vi "例程06-初级计算器.vi"() -> ()   [LabVIEW 2018]
panel:
  in  "/":bool
  in  "*":bool
  in  "-":bool
  in  "+":bool
  out "结果":dbl
  in  "输入2":dbl
  in  "输入1":dbl
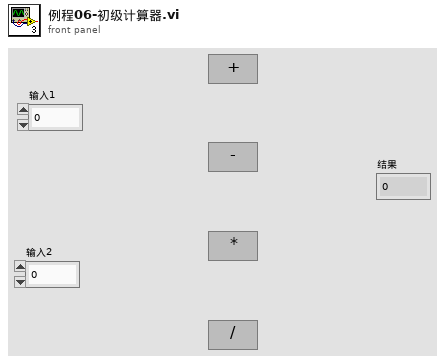
[diagram p1: front panel]
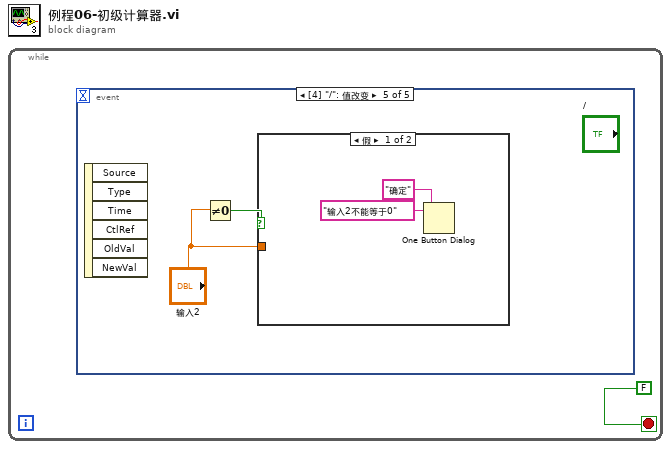
[diagram p0: block diagram]
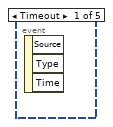
[diagram p2: hidden frame]
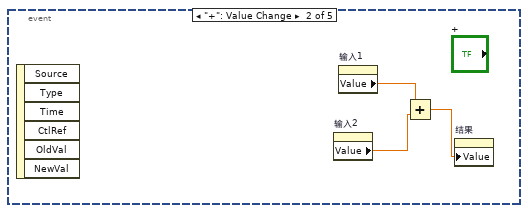
[diagram p3: hidden frame]
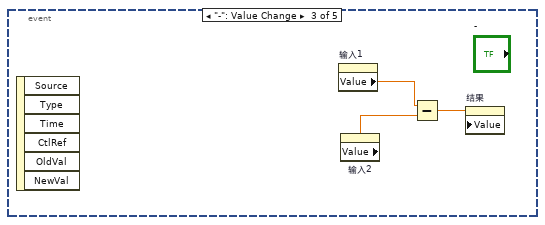
[diagram p4: hidden frame]
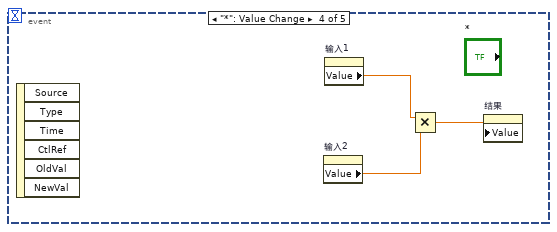
[diagram p5: hidden frame]
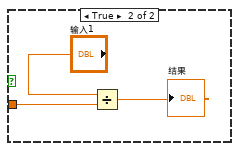
[diagram p6: hidden frame]
diagram:
  n1 = while {
    stop <- FALSE stop-if-true
    n2 = event shown="[4] \"/\": 值改变" {
      selector: _ -> [_ _ _ _ _]
      dyn-events: _ -> [_ _ _ _ _]
      timeout: _ -> [_ _ _ _ _]
      event Timeout {
        n3 = event-data() -> ()  [unwired: 1 in, 3 out]
      }
      event "+": Value Change {
        n4 = event-data() -> ()  [unwired: 1 in, 6 out]
        n5 = property on="输入2" class="DigNum (严格)"() -> ("Value"=w3:dbl)  [unwired: 2 in, 2 out]
        n6 = property on="输入1" class="DigNum (严格)"() -> ("Value"=w4:dbl)  [unwired: 2 in, 2 out]
        n7 = Add(x=w4, y=w3) -> (x+y=w2:dbl)
        n8 = property on="结果" class="DigNum (严格)"("Value"=w2) -> ()  [unwired: 2 in, 2 out]
      }
      event "-": Value Change {
        n9 = event-data() -> ()  [unwired: 1 in, 6 out]
        n10 = property on="输入1" class="DigNum (严格)"() -> ("Value"=w7:dbl)  [unwired: 2 in, 2 out]
        n11 = property on="输入2" class="DigNum (严格)"() -> ("Value"=w6:dbl)  [unwired: 2 in, 2 out]
        n12 = Subtract(x=w7, y=w6) -> (x-y=w5:dbl)
        n13 = property on="结果" class="DigNum (严格)"("Value"=w5) -> ()  [unwired: 2 in, 2 out]
      }
      event "*": Value Change {
        n14 = event-data() -> ()  [unwired: 1 in, 6 out]
        n15 = property on="输入2" class="DigNum (严格)"() -> ("Value"=w9:dbl)  [unwired: 2 in, 2 out]
        n16 = property on="输入1" class="DigNum (严格)"() -> ("Value"=w10:dbl)  [unwired: 2 in, 2 out]
        n17 = Multiply(x=w10, y=w9) -> (x*y=w8:dbl)
        n18 = property on="结果" class="DigNum (严格)"("Value"=w8) -> ()  [unwired: 2 in, 2 out]
      }
      event "/": Value Change {
        n19 = event-data() -> ()  [unwired: 1 in, 6 out]
        n20 = Not Equal To 0?(x="输入2") -> (x != 0?=w11:bool)
        n21 = case shown="假" w11 {
          tunnel: "输入2" -> [_ w16]
          frame False {
            n22 = One Button Dialog(message="输入2不能等于0" ("消息"), button name ("OK")="确定" ("按钮名称（“确定”）")) -> ()  [unwired: 1 out]
          }
          frame True {
            n23 = Divide(x="输入1", y=w16) -> (x/y=→"结果":dbl)
          }
        }
      }
    }
  }
